vi "DHE_write_tp.vi"(0 "fd":i32, 1 "board":string, 2 "memory":string, 3 "address":i32, 9 "value":string, 11 "error in (no error)":errorcluster, 12 "name":string, 13 "type":string) -> (4 "fd out":i32, 8 "return value":string, 10 "busy":bool, 15 "error out":errorcluster)   [LabVIEW 2016]
doc: "This VI closes the I/O interface with the instrument."
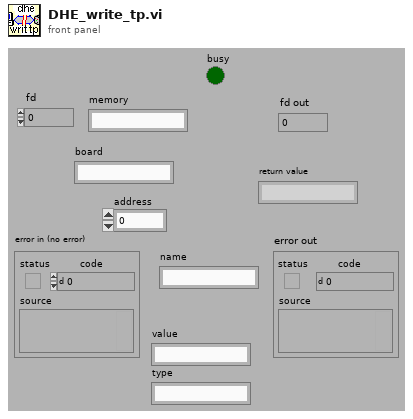
[diagram p1: front panel]
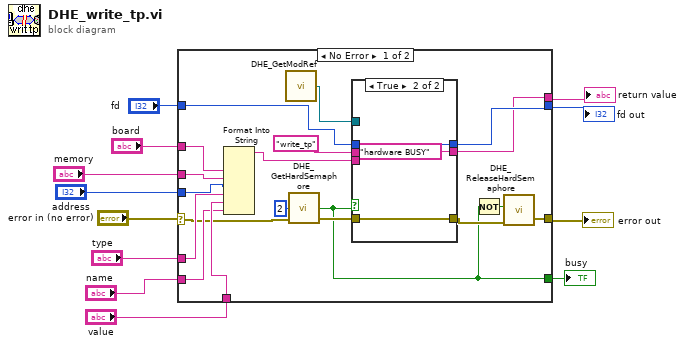
[diagram p0: block diagram]
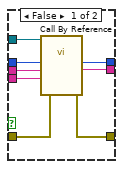
[diagram p2: hidden frame]
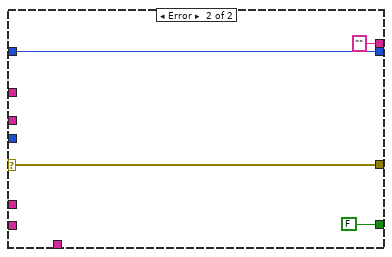
[diagram p3: hidden frame]
diagram:
  n1 = case shown="No Error" "error in (no error)" {
    selector: "error in (no error)" -> [w19 w45]
    tunnel: "fd" -> [w29 w46]
    tunnel: [w23 "" ("str result")] -> w11
    tunnel: [w15 w45] -> w10
    tunnel: [w28 w46] -> w9
    tunnel: "board" -> [w27 _]
    tunnel: "memory" -> [w26 _]
    tunnel: "address" -> [w25 _]
    tunnel: "type" -> [w22 _]
    tunnel: "name" -> [w20 _]
    tunnel: "value" -> [w21 _]
    tunnel: [w14 FALSE ("timed out")] -> w1
    frame No Error {
      n2 = Format Into String(w27, w26, w25, w22, w21, w20) -> (resulting string=w24:string)  [unwired: 3 in, 1 out]
      n3 = call "DHE_GetModRef.vi"() -> ("DHE_ModRef"=w31:refnum<vi>)  [unwired: 9 out]
      n4 = call "DHE_GetHardSemaphore.vi"("timeout"=2, "error in (no error)"=w19) -> ("timed out"=w14:bool, "error out"=w18:errorcluster)  [unwired: 6 out]
      n5 = case shown="True" w14 {
        tunnel: w31 -> [w39 _]
        tunnel: "write_tp" ("function") -> [w38 _]
        tunnel: w29 -> [w37 w42]
        tunnel: [w36 w42] -> w28
        tunnel: w24 -> [w35 _]
        tunnel: [w34 "hardware BUSY" ("str result")] -> w23
        tunnel: w18 -> [w33 w41]
        tunnel: [w32 w41] -> w16
        frame False {
          n6 = call-by-ref "?"(reference=w39, "error in (no error)"=w33, "arguments"=w35, "function"=w38, "fd in"=w37) -> ("error out"=w32:errorcluster, "str result"=w34:string, "fd out"=w36:i32)  [unwired: 5 in, 3 out]
        }
        frame True {
        }
      }
      n7 = Not(x=w14) -> (.not. x?=w13:bool)
      n8 = call "DHE_ReleaseHardSemaphore.vi"("error in (no error)"=w16, "release?"=w13) -> ("error out"=w15:errorcluster)  [unwired: 9 out]
    }
    frame Error {
    }
  }
  "error out" <- w10
  "return value" <- w11
  "fd out" <- w9
  "busy" <- w1
